vi "Testa_Leaf.vi"(9 "enable":bool, 11 "LEAF":i32) -> ()   [LabVIEW 2018]
uses:
  Global_Telescopio.vi
panel:
  out "error out 4":errorcluster
  out "error out 3":errorcluster
  out "error out 2":errorcluster
  out "concatenated string":string
  out "error out":errorcluster
  out "vi reference":refnum<vi>
  out "timeout":timestamp
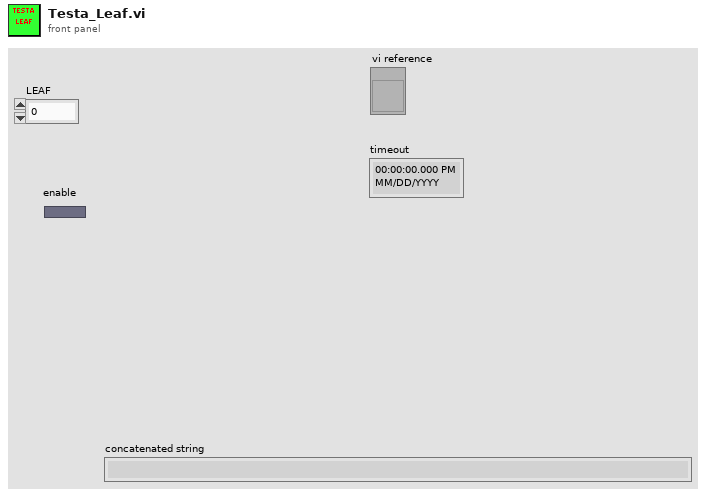
[diagram p1: front panel]
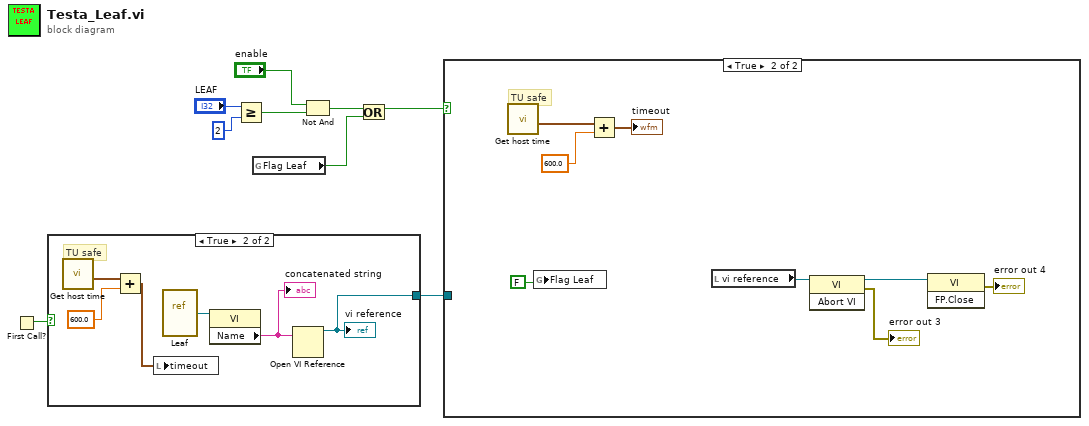
[diagram p0: block diagram]
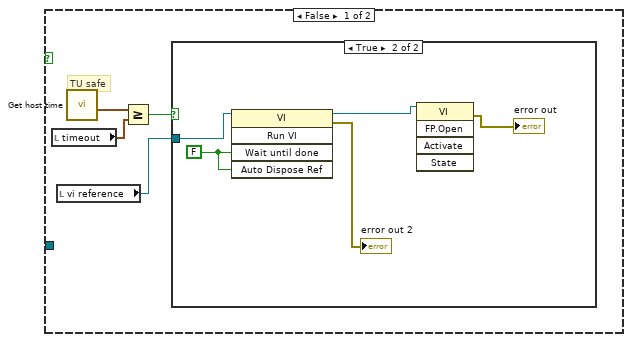
[diagram p3: hidden frame]
diagram:
  n1 = First Call?() -> (First Call?: T/F=w9:bool)
  n2 = case shown="True" w9 {
    tunnel: [_ w13] -> w8
    frame False {
    }
    frame True {
      # "TU safe"
      n3 = call "Get host time.vi"() -> ("BR current time"=w10:timestamp)  [unwired: 8 in, 3 out]
      n4 = Add(x=w10, y=600.0) -> (x+y=w11:timestamp)
      n5 = local write "timeout"(w11) -> ()
      n6 = vi-ref "Leaf.vi"() -> (w15:refnum<vi>)
      n7 = property class="VI"(reference=w15) -> ("Name"=w14:string)  [unwired: 1 in, 2 out]
      "concatenated string" <- w14
      n8 = Open VI Reference(vi path=w14) -> (vi reference=w13:refnum<vi>)  [unwired: 5 in, 1 out]
      "vi reference" <- w13
    }
  }
  n9 = Greater Or Equal?(x="LEAF", y=2) -> (x >= y?=w5:bool)
  n10 = global read "Global_Telescopio.vi" "Flag Leaf"() -> (w2:bool)
  n11 = Not And(1:w5, 2:"enable") -> (0:w4:bool)
  n12 = Or(x=w4, y=w2) -> (x .or. y?=w3:bool)
  n13 = case shown="True" w3 {
    tunnel: w8 -> [_ _]
    frame False {
      # "TU safe"
      n14 = local read "timeout"() -> (w19:timestamp)
      n15 = local read "vi reference"() -> (w18:refnum<vi>)
      n16 = call "Get host time.vi"() -> ("BR current time"=w16:timestamp)  [unwired: 8 in, 3 out]
      n17 = Greater Or Equal?(x=w16, y=w19) -> (x >= y?=w17:bool)
      n18 = case shown="True" w17 {
        tunnel: w18 -> [_ w23]
        frame False {
        }
        frame True {
          w24 = FALSE ("Wait Until Done")
          n19 = invoke class="VI" method="Run VI"(reference=w23, "Wait until done"=w24, "Auto Dispose Ref"=w24) -> (reference out=w22:refnum<vi>, error out=→"error out 2":errorcluster)  [unwired: 2 in, 3 out]
          n20 = invoke class="VI" method="FP.Open"(reference=w22) -> (error out=→"error out":errorcluster)  [unwired: 4 in, 4 out]
        }
      }
    }
    frame True {
      # "TU safe"
      n21 = call "Get host time.vi"() -> ("BR current time"=w25:timestamp)  [unwired: 8 in, 3 out]
      n22 = global write "Global_Telescopio.vi" "Flag Leaf"(FALSE) -> ()
      n23 = Add(x=w25, y=600.0) -> (x+y=→"timeout":timestamp)
      n24 = local read "vi reference"() -> (w28:refnum<vi>)
      n25 = invoke class="VI" method="Abort VI"(reference=w28) -> (reference out=w30:refnum<vi>, error out=→"error out 3":errorcluster)  [unwired: 2 in, 1 out]
      n26 = invoke class="VI" method="FP.Close"(reference=w30) -> (error out=→"error out 4":errorcluster)  [unwired: 2 in, 2 out]
    }
  }
